vi "test Peer-To-Peer Function Code Typedef.vi"(11 "Test Case In":refnum<class "Function Code Typedef Test.lvclass">) -> (0 "error out":errorcluster, 3 "Test Case Out":refnum<class "Function Code Typedef Test.lvclass">)   [LabVIEW 2020, in "Function Code Typedef Test.lvclass"]
uses:
  Function Code Typedef Test.lvclass
  Function Code Typedef Test.lvclass/Function Code Typedef Test.ctl
  C:/Program Files/National Instruments/LabVIEW 2026/vi.lib/Astemes/LUnit/Test Case.lvclass
  C:/Program Files/National Instruments/LabVIEW 2026/vi.lib/Astemes/LUnit/LUnit Runnable.lvclass
  D:/git/CANopen-LabVIEW/Tests/Function Code Typedef Test/Function Code Typedef Test.lvclass
  4993e8ee-a06a-463a-9684-69129f64d5ce.vi
  CANopen/Peer-To-Peer Function Code.ctl
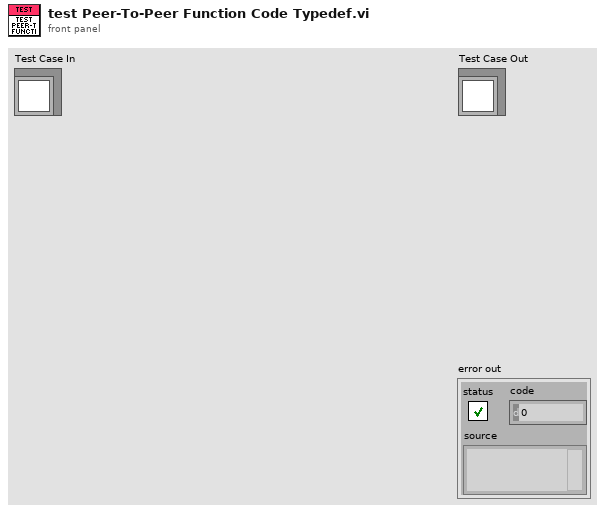
[diagram p1: front panel]
types:
  T1 = typedef "CANopen.lvlib/CANopen.lvclass/Peer-To-Peer Function Code.ctl" = map{string, i32}
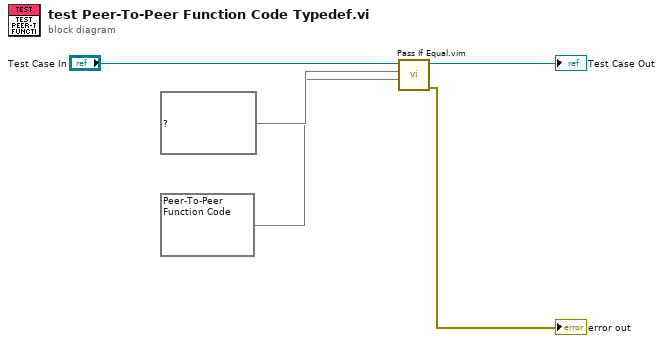
[diagram p0: block diagram]
diagram:
  n1 = call "Pass If Equal.vim"("Actual"=T1 {"EMCY"=1, "NMT Error Control"=14, "PDO1 (rx)"=4, "PDO1 (tx)"=3, "PDO2 (rx)"=6, "PDO2 (tx)"=5, "PDO3 (rx)"=8, "PDO3 (tx)"=7, "PDO4 (rx)"=10, "PDO4 (tx)"=9, "SDO (rx)"=12, "SDO (tx)"=11} ("Peer-2-Peer Function Code"), "Expected"=map{string, i32} {"EMCY"=1, "NMT Error Control"=14, "PDO1 (rx)"=4, "PDO1 (tx)"=3, "PDO2 (rx)"=6, "PDO2 (tx)"=5, "PDO3 (rx)"=8, "PDO3 (tx)"=7, "PDO4 (rx)"=10, "PDO4 (tx)"=9, "SDO (rx)"=12, "SDO (tx)"=11} ("Peer-2-Peer Function Code"), "LUnit Test Case In"="Test Case In") -> ("error out"=→"error out":errorcluster, "LUnit Test Case Out"=→"Test Case Out":refnum<class "Function Code Typedef Test.lvclass">)  [unwired: 7 in]
